vi "ErrorViewer.Example.vi"() -> ()   [LabVIEW 2024]
uses:
  ErrorViewer.lvclass
  C:/Git/JA/JQMH/RQMHCore/ModuleCore/Module.lvclass
  RQMHCore/ErrorReporting/LogHandle/Event/EventLogHandle.lvclass/EventLogHandle.ctl
  RQMHCore/ErrorReporting/Record/LogRecord.lvclass
  RQMHCore/ErrorReporting/LogHandle/Event/EventLogHandle.lvclass
  C:/Git/JA/JQMH/ModuleTemplates/ErrorViewer/ErrorViewer.lvclass
  RQMHCore/Startup/ModuleStartup.lvclass
  RQMHCore/ModuleCore/Module.lvclass
  RQMHCore/ModuleCore/Show Front Panel.vi
  RQMHCore/ErrorReporting/Shared/Level.ctl
  RQMHCore/ErrorReporting/Shared/LoggerShared.lvlib
panel:
  in  "stop":bool
  out "error out":errorcluster
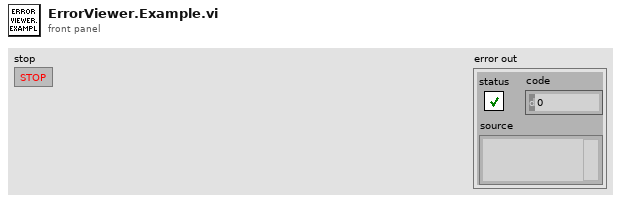
[diagram p1: front panel]
types:
  T1 = typedef "LoggerShared.lvlib/Level.ctl" = enum16{"DEBUG", "INFO", "WARNING", "ERROR", "CRITICAL"}
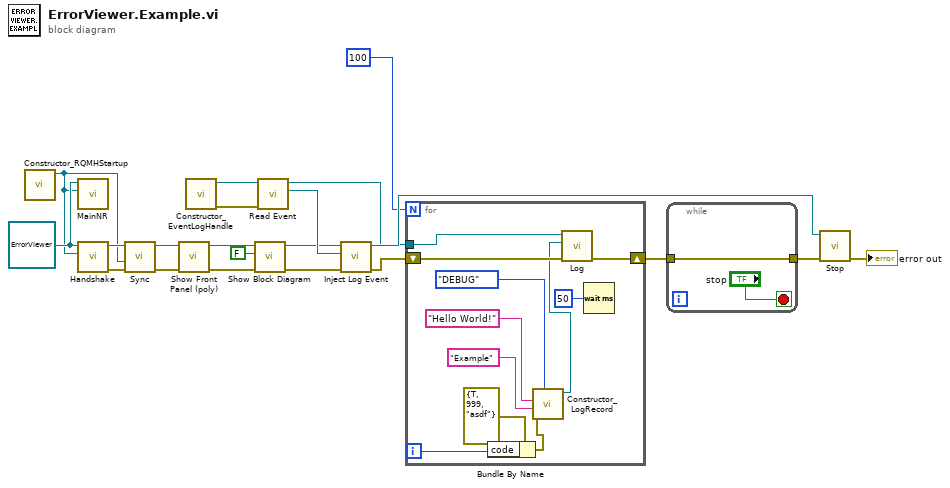
[diagram p0: block diagram]
diagram:
  w16 = refnum<class "ErrorViewer.lvclass"> refnum ("Template")
  n1 = call "Constructor_RQMHStartup.vi"() -> ("JQMHStartup out"=w15:refnum<class "ModuleStartup.lvclass">)  [unwired: 10 in, 1 out]
  n2 = call-dynamic "MainNR.vi"("JQMHStartup"=w15, "ErrorViewer in"=w16) -> ()  [unwired: 10 in]
  n3 = call "Handshake.vi"("JQMHStartup in"=w15, "JQMHModule in"=w16) -> ("error out"=w20:errorcluster, "JQMHModule out"=w21:refnum<class "ErrorViewer.lvclass">)  [unwired: 7 in, 1 out]
  n4 = call "Sync.vi"("error in (no error)"=w20, "StartupHandshake out"=w15, "JQMHCore in"=w21) -> ("error out"=w18:errorcluster, "JQMHCore out"=w19:refnum<class "ErrorViewer.lvclass">)  [unwired: 7 in]
  n5 = call-poly "Show Front Panel (poly).vi"("error in (no error)"=w18, "JQMHCore in"=w19) -> ("error out"=w11:errorcluster, "JQMHCore out"=w5:refnum<class "ErrorViewer.lvclass">)  [unwired: 8 in]
  n6 = call "Constructor_EventLogHandle.vi"() -> ("error out"=w13:errorcluster, "EventHandle"=w14:refnum<class "EventLogHandle.lvclass">)  [unwired: 10 in]
  n7 = call "Show Block Diagram.vi"("error in (no error)"=w11, "For Debug? (T)"=FALSE, "JQMHCore in"=w5) -> ("error out"=w6:errorcluster, "JQMHCore out"=w4:refnum<class "ErrorViewer.lvclass">)  [unwired: 7 in]
  n8 = call "Read Event.vi"("error in (no error)"=w13, "EventLogHandle in"=w14) -> ("Event"=w10:refnum<user-event>, "EventLogHandle out"=w9:refnum<class "EventLogHandle.lvclass">)  [unwired: 7 in, 1 out]
  n9 = call "Inject Log Event.vi"("error in (no error)"=w6, "Log Event"=w10, "NewTemplate in"=w4) -> ("error out"=w8:errorcluster, "NewTemplate out"=w12:refnum<class "ErrorViewer.lvclass">)  [unwired: 6 in, 1 out]
  n10 = for {
    N: 100 -> [_]
    tunnel: w9 -> [w32]
    shift-right: [w29] -> w3
    shift-left: w8 -> [w31]
    i -> [w23]
    n11 = Bundle By Name(cluster=errorcluster {"status"=TRUE, "code"=999, "source"="asdf"} ("Error to log"), "code"=w23) -> (w22:errorcluster)
    n12 = call "Constructor_LogRecord.vi"("Level"=Level."DEBUG", "Error to log"=w22, "Source"="Example", "Message"="Hello World!") -> ("LogRecord out"=w24:refnum<class "LogRecord.lvclass">)  [unwired: 7 in]
    n13 = call-dynamic "Log.vi"("error in (no error)"=w31, "LogRecord"=w24, "EventLogHandle in"=w32) -> ("error out"=w29:errorcluster)  [unwired: 7 in, 1 out]
    n14 = Wait (ms)(milliseconds to wait=u32 50) -> ()  [unwired: 1 out]
  }
  n15 = while {
    tunnel: w3 -> [w33]
    tunnel: [w33] -> w2
    stop <- "stop" stop-if-true
  }
  n16 = call "Stop.vi"("error in (no error)"=w2, "JQMHCore in"=w12) -> ("error out"=→"error out":errorcluster)  [unwired: 9 in]
